vi "make-Lines.vi"(6 "Shutter off between lines":bool, 7 "Slide in":refnum<vi>, 8 "error in":errorcluster, 9 "d (um)":dbl=1.0, 10 "L (um)":dbl=20.0, 11 "N Lines":i32=20) -> (0 "error out":errorcluster, 3 "Progress":i32=65)   [LabVIEW 2014]
doc: "André Romero - 2023\nandretec@ifsc.usp.br\nIFSC - USP"
uses:
  Global Motors.vi
panel:
  out "Progress (%)":u8(slide)=100 scale=0.0..100.0
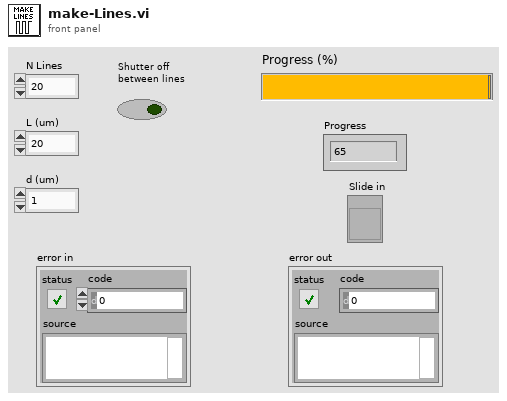
[diagram p1: front panel]
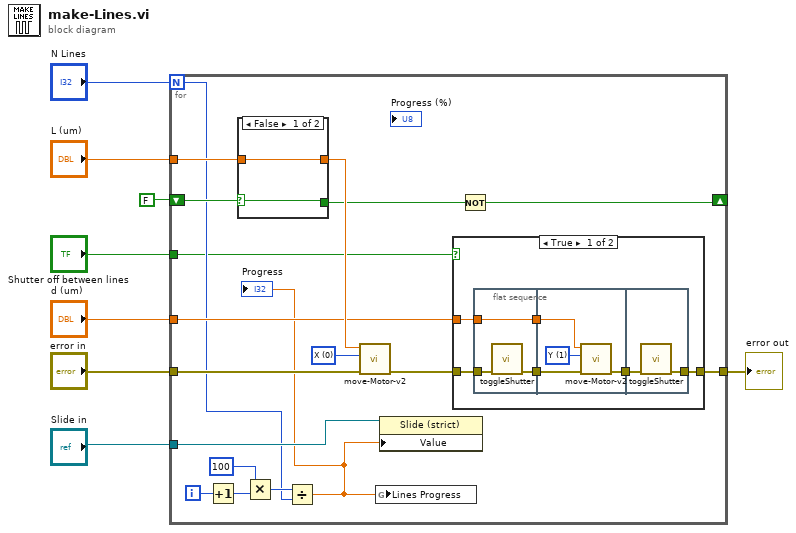
[diagram p0: block diagram]
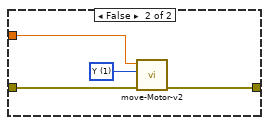
[diagram p2: hidden frame]
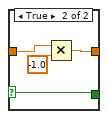
[diagram p3: hidden frame]
diagram:
  n1 = for {
    N: "N Lines" -> [w11]
    tunnel: "error in" -> [w25]
    tunnel: "L (um)" -> [w22]
    shift-right: [w19] -> _
    shift-left: FALSE -> [w23]
    tunnel: "d (um)" -> [w18]
    tunnel: [w17] -> w8
    tunnel: "Slide in" -> [w15]
    tunnel: "Shutter off between lines" -> [w9]
    i -> [w16]
    w26 = u16 0 items=["X", "Y"] ("Axis")
    n2 = Increment(x=w16) -> (x+1=w14:i32)
    n3 = case shown="False" w23 {
      selector: w23 -> [w46 w48]
      tunnel: w22 -> [w47 w49]
      tunnel: [w47 w51] -> w21
      tunnel: [w46 w48] -> w20
      frame False {
      }
      frame True {
        n4 = Multiply(x=w49, y=-1.0) -> (x*y=w51:dbl)
      }
    }
    n5 = Multiply(x=100, y=w14) -> (x*y=w12:i32)
    n6 = Divide(x=w12, y=w11) -> (x/y=w10:dbl)
    "Progress" <- w10
    n7 = call "move-Motor-v2.vi"("error in"=w25, "Axis"=w26, "Distance (um)"=w21) -> ("error out"=w24:errorcluster)  [unwired: 8 in]
    n8 = global write "Global Motors.vi" "Lines Progress"(w10) -> ()
    n9 = property class="Slide (strict)"(reference=w15, "Value"=w10) -> ()  [unwired: 1 in, 2 out]
    n10 = case shown="True" w9 {
      tunnel: w24 -> [w32 w44]
      tunnel: w18 -> [w31 w43]
      tunnel: [w30 w42] -> w17
      frame True {
        n11 = flat-sequence {
          tunnel: w31 -> [w35]
          tunnel: w32 -> [w34]
          tunnel: [w35] -> w29
          tunnel: [w33] -> w27
          tunnel: w29 -> [w37]
          tunnel: [w36] -> w28
          tunnel: w27 -> [w38]
          tunnel: [w40] -> w30
          tunnel: w28 -> [w41]
          frame #0 {
            n12 = call "toggleShutter.vi"("Error In"=w34) -> ("error out"=w33:errorcluster)  [unwired: 9 in]
          }
          frame #1 {
            w39 = u16 1 items=["X", "Y"] ("Axis")
            n13 = call "move-Motor-v2.vi"("error in"=w38, "Axis"=w39, "Distance (um)"=w37) -> ("error out"=w36:errorcluster)  [unwired: 8 in]
          }
          frame #2 {
            n14 = call "toggleShutter.vi"("Error In"=w41) -> ("error out"=w40:errorcluster)  [unwired: 9 in]
          }
        }
      }
      frame False {
        w45 = u16 1 items=["X", "Y"] ("Axis")
        n15 = call "move-Motor-v2.vi"("error in"=w44, "Axis"=w45, "Distance (um)"=w43) -> ("error out"=w42:errorcluster)  [unwired: 8 in]
      }
    }
    n16 = Not(x=w20) -> (.not. x?=w19:bool)
  }
  "error out" <- w8
